vi "Gantry Demonstration.vi"() -> ()   [LabVIEW 2017]
uses:
  Shared Components/Gantry Class/Gantry Class.lvclass
  Shared Components/Gantry Class/Type Definitions/Init_Modes.ctl
  Shared Components/WorkTable Class/Type Definitions/Worktable_Mode.ctl
  Shared Components/Vec3d Class/Vec3d Class.lvclass
  Shared Components/Gantry Class/Type Definitions/Virtual Modes.ctl
panel:
  out "error out":errorcluster
  in  "Config Folder":path=path "C:/Users/husker/Desktop/gantry/Config"
  in  "Virtual Mode":T1
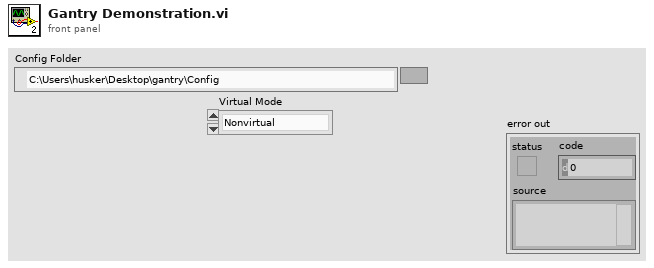
[diagram p1: front panel]
types:
  T1 = typedef "Virtual Modes.ctl" = enum16{"Nonvirtual", "Virtual"}
  T2 = typedef "Worktable_Mode.ctl" = enum16{"Encapsulation", "Gluing"}
  T3 = typedef "Init_Modes.ctl" = enum16{"Full", "Robot Only", "Dispenser Only", "Cameras Only", "Robot and Cameras", "Robot and Cameras and Dispenser", "Manifold Only"}
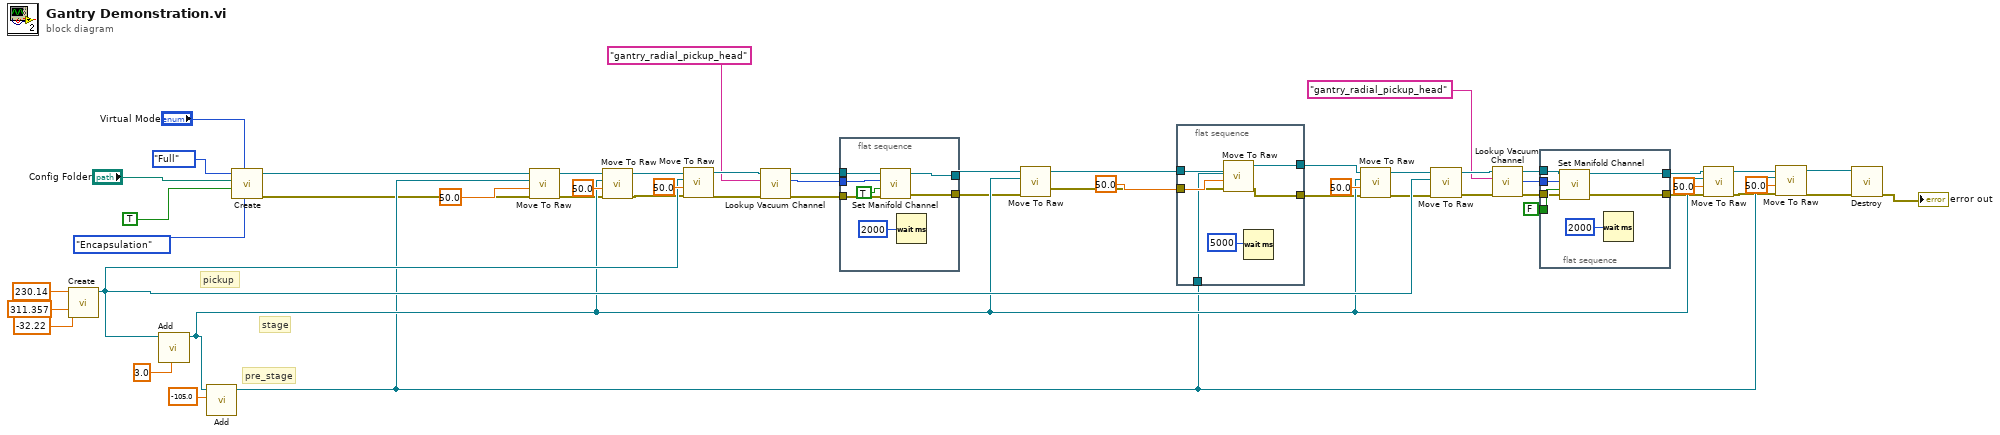
[diagram p0: block diagram]
diagram:
  # "pre_stage"
  # "stage"
  # "pickup"
  n1 = call "Create.vi"("Z"=-32.22, "Y"=311.357, "X"=230.14) -> ("Vec3d Class out"=w27:refnum<class "Vec3d Class.lvclass">)  [unwired: 7 in, 1 out]
  n2 = call-dynamic "Add.vi"("Z"=3.0, "Vec3d in"=w27) -> ("Vec3d out"=w20:refnum<class "Vec3d Class.lvclass">)  [unwired: 7 in, 1 out]
  n3 = call-dynamic "Add.vi"("X"=-105.0, "Vec3d in"=w20) -> ("Vec3d out"=w17:refnum<class "Vec3d Class.lvclass">)  [unwired: 7 in, 1 out]
  n4 = call "Create.vi"(6:Worktable_Mode."Encapsulation" ("Worktable Mode"), "Virtual Mode"="Virtual Mode", "HOME?"=TRUE, "Config Folder"="Config Folder", "Init Mode"=Init_Modes."Full") -> ("error out"=w1:errorcluster, "Gantry out"=w43:refnum<class "Gantry Class.lvclass">)  [unwired: 5 in]
  n5 = call-dynamic "Move To Raw.vi"("error in"=w1, "Speed"=50.0, "Destination"=w17, "Gantry in"=w43) -> ("error out"=w2:errorcluster, "Gantry out"=w41:refnum<class "Gantry Class.lvclass">)  [unwired: 6 in]
  n6 = call-dynamic "Move To Raw.vi"("error in"=w2, "Speed"=50.0, "Destination"=w20, "Gantry in"=w41) -> ("error out"=w3:errorcluster, "Gantry out"=w39:refnum<class "Gantry Class.lvclass">)  [unwired: 6 in]
  n7 = call-dynamic "Move To Raw.vi"("error in"=w3, "Speed"=50.0, "Destination"=w27, "Gantry in"=w39) -> ("error out"=w4:errorcluster, "Gantry out"=w37:refnum<class "Gantry Class.lvclass">)  [unwired: 6 in]
  n8 = call-dynamic "Lookup Vacuum Channel.vi"("error in (no error)"=w4, "Channel Name"="gantry_radial_pickup_head" ("String"), "Gantry Class in"=w37) -> ("error out"=w5:errorcluster, "Channel Number"=w35:i32, "Gantry Class out"=w34:refnum<class "Gantry Class.lvclass">)  [unwired: 5 in]
  n9 = flat-sequence {
    tunnel: w35 -> [w60]
    tunnel: w34 -> [w59]
    tunnel: [w57] -> w33
    tunnel: [w56] -> w6
    tunnel: w5 -> [w55]
    frame #0 {
      n10 = call-dynamic "Set Manifold Channel.vi"("error in"=w55, "On/Off"=TRUE, "Manifold Channel"=w60, "Gantry in"=w59) -> ("error out"=w56:errorcluster, "Gantry out"=w57:refnum<class "Gantry Class.lvclass">)  [unwired: 6 in]
      n11 = Wait (ms)(milliseconds to wait=u32 2000) -> ()  [unwired: 1 out]
    }
  }
  n12 = call-dynamic "Move To Raw.vi"("error in"=w6, "Destination"=w20, "Gantry in"=w33) -> ("error out"=w7:errorcluster, "Gantry out"=w31:refnum<class "Gantry Class.lvclass">)  [unwired: 7 in]
  n13 = flat-sequence {
    tunnel: 50.0 ("Speed") -> [w68]
    tunnel: w17 -> [w67]
    tunnel: w31 -> [w66]
    tunnel: [w65] -> w30
    tunnel: [w63] -> w8
    tunnel: w7 -> [w62]
    frame #0 {
      n14 = call-dynamic "Move To Raw.vi"("error in"=w62, "Speed"=w68, "Destination"=w67, "Gantry in"=w66) -> ("error out"=w63:errorcluster, "Gantry out"=w65:refnum<class "Gantry Class.lvclass">)  [unwired: 6 in]
      n15 = Wait (ms)(milliseconds to wait=u32 5000 ("millisecond timer value")) -> ()  [unwired: 1 out]
    }
  }
  n16 = call-dynamic "Move To Raw.vi"("error in"=w8, "Speed"=50.0, "Destination"=w20, "Gantry in"=w30) -> ("error out"=w9:errorcluster, "Gantry out"=w28:refnum<class "Gantry Class.lvclass">)  [unwired: 6 in]
  n17 = call-dynamic "Move To Raw.vi"("error in"=w9, "Destination"=w27, "Gantry in"=w28) -> ("error out"=w10:errorcluster, "Gantry out"=w26:refnum<class "Gantry Class.lvclass">)  [unwired: 7 in]
  n18 = call-dynamic "Lookup Vacuum Channel.vi"("error in (no error)"=w10, "Channel Name"="gantry_radial_pickup_head" ("String"), "Gantry Class in"=w26) -> ("error out"=w11:errorcluster, "Channel Number"=w22:i32, "Gantry Class out"=w24:refnum<class "Gantry Class.lvclass">)  [unwired: 5 in]
  n19 = flat-sequence {
    tunnel: w24 -> [w75]
    tunnel: FALSE ("On/Off") -> [w74]
    tunnel: w22 -> [w73]
    tunnel: [w71] -> w21
    tunnel: [w70] -> w12
    tunnel: w11 -> [w69]
    frame #0 {
      n20 = call-dynamic "Set Manifold Channel.vi"("error in"=w69, "On/Off"=w74, "Manifold Channel"=w73, "Gantry in"=w75) -> ("error out"=w70:errorcluster, "Gantry out"=w71:refnum<class "Gantry Class.lvclass">)  [unwired: 6 in]
      n21 = Wait (ms)(milliseconds to wait=u32 2000) -> ()  [unwired: 1 out]
    }
  }
  n22 = call-dynamic "Move To Raw.vi"("error in"=w12, "Speed"=50.0, "Destination"=w20, "Gantry in"=w21) -> ("error out"=w13:errorcluster, "Gantry out"=w18:refnum<class "Gantry Class.lvclass">)  [unwired: 6 in]
  n23 = call-dynamic "Move To Raw.vi"("error in"=w13, "Speed"=50.0, "Destination"=w17, "Gantry in"=w18) -> ("error out"=w14:errorcluster, "Gantry out"=w15:refnum<class "Gantry Class.lvclass">)  [unwired: 6 in]
  n24 = call "Destroy.vi"("error in"=w14, "Gantry Class in"=w15) -> ("error out"=→"error out":errorcluster)  [unwired: 9 in]
